vi "getTime.vi"() -> (0 "Current Time":string)   [LabVIEW 2010]
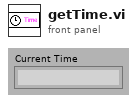
[diagram p1: front panel]
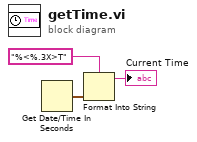
[diagram p0: block diagram]
diagram:
  n1 = Get Date/Time In Seconds() -> (seconds since 1Jan1904=w1:timestamp)
  n2 = Format Into String(format string="%<%.3X>T", w1) -> (resulting string=→"Current Time":string)  [unwired: 2 in, 1 out]
